vi "setActorParametersJson.vi"(8 "error":errorcluster, 9 "json_dict":string, 10 "axis":i32, 11 "connection ID":refnum<k5>) -> (0 "error out":errorcluster, 2 "axis_out":i32, 3 "connection ID out":refnum<k5>)   [LabVIEW 2016, in "amc_api.lvlib"]
doc: "This function can be used to change several actor parameters with one call."
uses:
  amc_api.lvlib
panel:
  out "jsonRespIn":string
  out "JSON-response":string="{\"jsonrpc\":\"2.0\",\"method\":\"\",\"params\":[5,1.245,true,\"name\"],\"id\":\"1\"}"
  out "JSON request":string
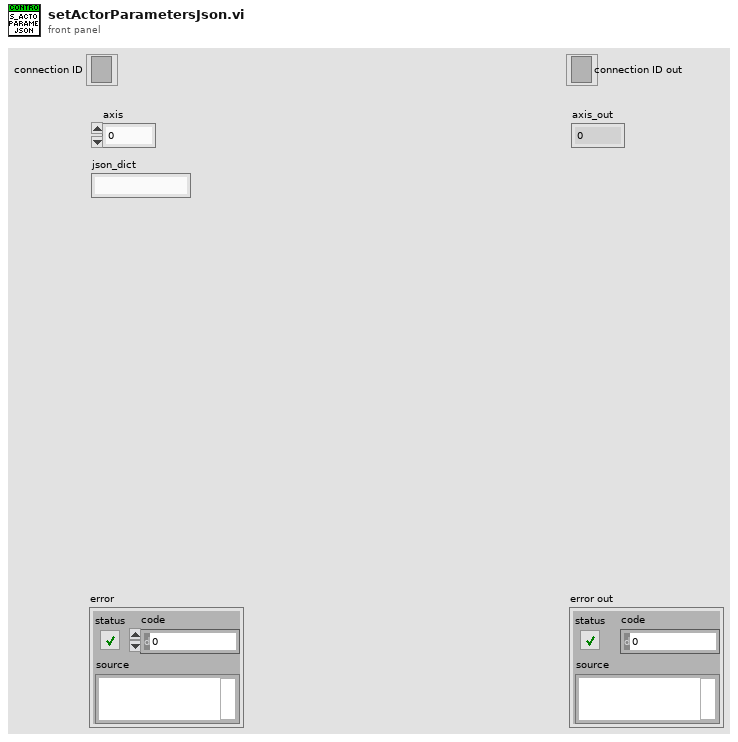
[diagram p1: front panel]
types:
  T1 = cluster{"jsonrpc":string, "method":string, "params":string[], "id":string, "api":i32, "pid":string}
  T2 = enum16{"Standard", "Buffered", "CRLF", "Immediate"}
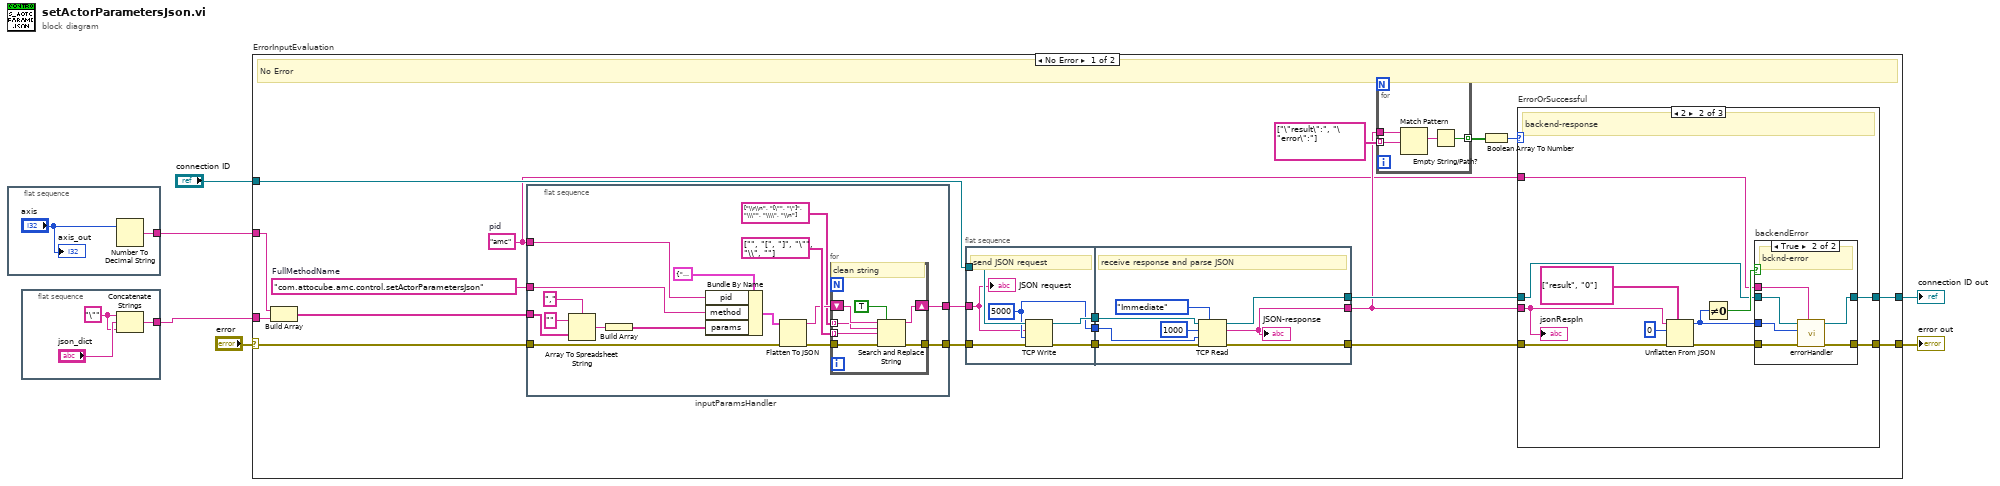
[diagram p0: block diagram]
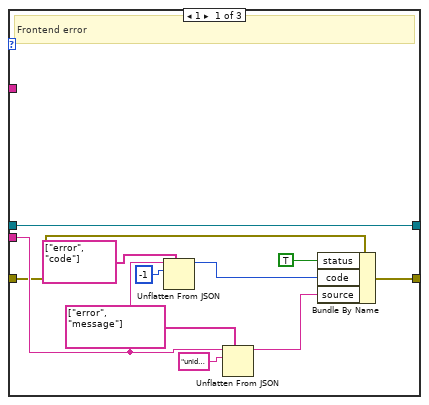
[diagram p2: hidden frame]
diagram:
  n1 = flat-sequence "in_axis" {
    tunnel: [w8] -> w2
    frame #0 {
      n2 = Number To Decimal String(number="axis") -> (decimal integer string=w8:string)  [unwired: 1 in]
      "axis_out" <- "axis"
    }
  }
  n3 = flat-sequence "in_string" {
    tunnel: [w10] -> w1
    frame #0 {
      w9 = "\"" ("string")
      n4 = Concatenate Strings(w9, "json_dict", w9) -> (w10:string)
    }
  }
  n5 = case "ErrorInputEvaluation" shown="No Error" "error" {
    selector: "error" -> [w18 w105]
    tunnel: "connection ID" -> [w28 w106]
    tunnel: [w20 w105] -> w5
    tunnel: [w21 w106] -> w4
    tunnel: w2 -> [w13 _]
    tunnel: w1 -> [w12 _]
    frame No Error {
      w14 = "amc"  # pid
      w19 = "com.attocube.amc.control.setActorParametersJson"  # FullMethodName
      # "No Error"
      n6 = Build Array ("ParametersArrayString")(w13, w12) -> (w17:string[])
      n7 = flat-sequence "inputParamsHandler" {
        tunnel: [w37] -> w16
        tunnel: w17 -> [w43]
        tunnel: w18 -> [w42]
        tunnel: [w39] -> w15
        tunnel: w19 -> [w33]
        tunnel: w14 -> [w32]
        frame #0 {
          n8 = Array To Spreadsheet String(delimiter (Tab)=",", array=w43, 3:"" ("format string")) -> (spreadsheet string=w45:string)
          n9 = Build Array "Build Array"(w45) -> (w34:string[])
          n10 = Bundle By Name(cluster=T1 {"jsonrpc"="2.0", "method"="com.attocube.amc.res.setRESReadOutFreq", "params"=[], "id"="1", "api"=2, "pid"=""}, "pid"=w32, "method"=w33, "params"=w34) -> (w44:T1)
          n11 = Flatten To JSON(anything=w44, error in (no error)=w42) -> (JSON string=w38:string, 11:w40:errorcluster)  [unwired: 1 in]
          n12 = for {
            tunnel: string[] ["\\r\\n", "[\"", "\"]", "\\\"", "\\\\", "\\n"] ("search string") -> [w51] mode=indexing
            tunnel: string[] ["", "[", "]", "\"", "\\", ""] ("replace string (\"\")") -> [w50] mode=indexing
            shift-right: [w53] -> w37
            shift-left: w38 -> [w52]
            tunnel: w40 -> [w49]
            tunnel: [w48] -> w39
            # "clean string"
            n13 = Search and Replace String(replace all?=TRUE ("replace all? (F)"), input string=w52, search string=w51, replace string=w50, error in=w49) -> (result string=w53:string, error out=w48:errorcluster)  [unwired: 3 in, 2 out]
          }
        }
      }
      n14 = flat-sequence {
        tunnel: w28 -> [w96]
        tunnel: [w94] -> w31
        tunnel: [w95] -> w30
        tunnel: w15 -> [w91]
        tunnel: [w93] -> w29
        tunnel: w16 -> [w92]
        tunnel: [w100] -> w24
        tunnel: w31 -> [w102]
        tunnel: w30 -> [w101]
        tunnel: [w98] -> w23
        tunnel: w29 -> [w99]
        tunnel: [w97] -> w22
        frame #0 {
          w93 = 5000 ("timeout ms (25000)")
          # "send JSON request"
          n15 = TCP Write(connection ID=w96, data in=w92, error in (no error)=w91, 9:w93) -> (connection ID out=w94:refnum<k5>, error out=w95:errorcluster)  [unwired: 1 out]
          "JSON request" <- w92
        }
        frame #1 {
          # "receive response and parse JSON"
          n16 = TCP Read(connection ID=w102, bytes to read=1000, error in (no error)=w101, 7:T2."Immediate" ("mode (standard)"), 9:w99) -> (connection ID out=w100:refnum<k5>, data out=w97:string, error out=w98:errorcluster)
          "JSON-response" <- w97
        }
      }
      n17 = for {
        tunnel: string[] ["\"result\":", "\"error\":"] ("path") -> [w57] mode=indexing
        tunnel: [w55] -> w26 mode=indexing
        tunnel: w22 -> [w58]
        n18 = Match Pattern(string=w58, regular expression=w57) -> (match substring=w56:string)  [unwired: 1 in, 3 out]
        n19 = Empty String/Path?(string/path=w56) -> (empty?=w55:bool)
      }
      n20 = Boolean Array To Number(Boolean array=w26) -> (number=w25:u32)
      n21 = case "ErrorOrSuccessful" shown="2" w25 {
        tunnel: w22 -> [w61 w71 _]
        tunnel: w24 -> [w59 w74 w90]
        tunnel: [w59 w73 w90] -> w21
        tunnel: [w62 w72 w89] -> w20
        tunnel: w23 -> [w60 w75 w89]
        tunnel: w14 -> [_ w70 _]
        frame 1 {
          # "Frontend error"
          n22 = Unflatten From JSON(path=string[] ["error", "code"], JSON string=w61, type and defaults=-1) -> (value=w68:i32)  [unwired: 4 in, 1 out]
          n23 = Unflatten From JSON(path=string[] ["error", "message"], JSON string=w61, type and defaults="unidentified error") -> (value=w69:string)  [unwired: 4 in, 1 out]
          n24 = Bundle By Name(cluster=w60, "status"=TRUE, "code"=w68, "source"=w69) -> (w62:errorcluster)
        }
        frame 2 {
          # "backend-response"
          n25 = Unflatten From JSON(path=string[] ["result", "0"], JSON string=w71, type and defaults=0, error in (no error)=w75) -> (value=w80:i32, error out=w78:errorcluster)  [unwired: 3 in]
          n26 = Not Equal To 0?(x=w80) -> (x != 0?=w79:bool)
          n27 = case "backendError" shown="True" w79 {
            tunnel: w80 -> [_ w88]
            tunnel: w78 -> [w82 w87]
            tunnel: [w81 w86] -> w73
            tunnel: [w82 w85] -> w72
            tunnel: w74 -> [w81 w84]
            tunnel: w70 -> [_ w83]
            frame False {
              # "successful"
            }
            frame True {
              # "bcknd-error"
              n28 = call "errorHandler.vi"("pid"=w83, "error in"=w87, "errNbr"=w88, "connection ID"=w84) -> ("error out 2"=w85:errorcluster, "connection ID out"=w86:refnum<k5>)  [unwired: 6 in]
            }
          }
          "jsonRespIn" <- w71
        }
        frame Default {
          # "NoResponse"
        }
      }
    }
    frame Error {
      # "Error"
    }
  }
  "error out" <- w5
  "connection ID out" <- w4
